vi "Test Run Suite of Several Suites.vi"(8 "error in (no error)":errorcluster, 11 "Test Case In":refnum<class "LUnit Test Suite Tests.lvclass">) -> (0 "error out":errorcluster, 3 "Test Case Out":refnum<class "LUnit Test Suite Tests.lvclass">)   [LabVIEW 2020, in "LUnit Test Suite Tests.lvclass"]
uses:
  LUnit Test Suite Tests.lvclass
  LUnit Test Suite Tests.lvclass/LUnit Test Suite Tests.ctl
  source/LUnit Test Suite.lvclass
  Test Doubles/Test Case Test Double Child/Light Test Case Double.lvclass
  C:/git/astemes-lunit/source/Core/Runnable/Runnable.lvclass
  Test Doubles/Light Test Case Double Copy/Light Test Case Double Copy.lvclass
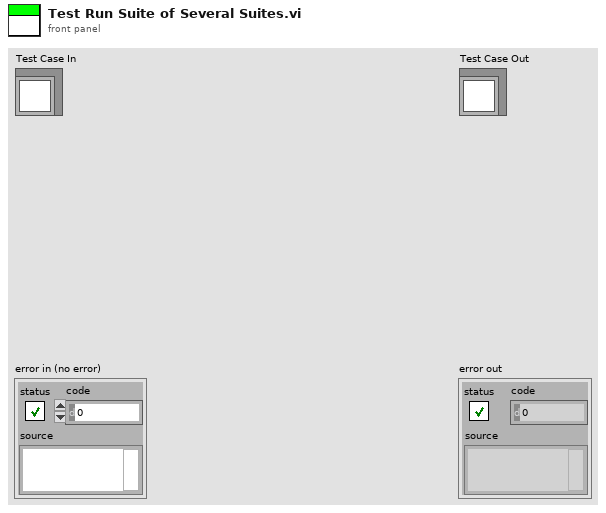
[diagram p1: front panel]
types:
  T1 = typedef "Result.lvlib/Result.ctl" = cluster{"Name":string, "Description":string, "Status":T2, "Result Type":T3, "Execution Time":dbl, "Data":cluster{"Expected":variant, "Actual":variant, "Delta":variant}}
  T2 = typedef "Result.lvlib/Status.ctl" = enum16{"", "Passed", "Failed", "Error", "Skipped", "Setup Error", "Broken", "Teardown Error"}
  T3 = typedef "Result.lvlib/Type.ctl" = enum16{"Test Case", "Test Suite", "Test Run", "Pass", "Fail", "Skip", "Pass if", "Fail if", "Pass if Error", "Fail if Error", "Pass if Equal", "Fail if Equal"}
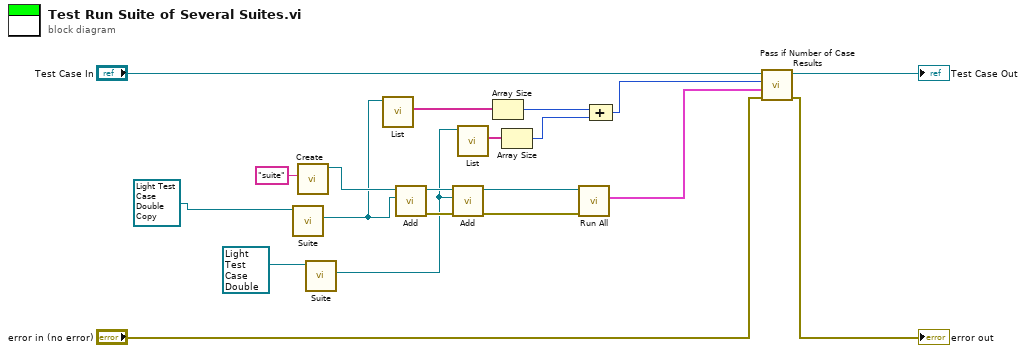
[diagram p0: block diagram]
diagram:
  n1 = call-dynamic "Suite.vi"("LUnit Test Case In"=refnum<class "Light Test Case Double Copy.lvclass"> refnum ("Light Test Case Double Copy.lvclass")) -> ("LUnit Test Suite Out"=w10:refnum<class "LUnit Test Suite.lvclass">)  [unwired: 8 in, 2 out]
  n2 = call "Create.vi"("Suite Name"="suite") -> ("LUnit Test Suite Out"=w11:refnum<class "LUnit Test Suite.lvclass">)  [unwired: 9 in, 1 out]
  n3 = call-dynamic "Suite.vi"("LUnit Test Case In"=refnum<class "Light Test Case Double.lvclass"> refnum ("Light Test Case Double.lvclass")) -> ("LUnit Test Suite Out"=w9:refnum<class "LUnit Test Suite.lvclass">)  [unwired: 8 in, 2 out]
  n4 = call "List.vi"("LUnit Test Suite In"=w10) -> ("List of Runnables"=w6:string[])  [unwired: 9 in, 1 out]
  n5 = call "Add.vi"("Runnable"=w10, "LUnit Test Suite In"=w11) -> ("error out"=w15:errorcluster, "LUnit Test Suite Out"=w14:refnum<class "LUnit Test Suite.lvclass">)  [unwired: 8 in]
  n6 = call "Add.vi"("error in (no error)"=w15, "Runnable"=w9, "LUnit Test Suite In"=w14) -> ("error out"=w16:errorcluster, "LUnit Test Suite Out"=w3:refnum<class "LUnit Test Suite.lvclass">)  [unwired: 7 in]
  n7 = call "List.vi"("LUnit Test Suite In"=w9) -> ("List of Runnables"=w8:string[])  [unwired: 9 in, 1 out]
  n8 = Array Size(array=w6) -> (size(s)=w5:i32)
  n9 = Array Size(array=w8) -> (size(s)=w7:i32)
  n10 = call "Run All.vi"("error in (no error)"=w16, "Runnable In"=w3) -> ("Results"=w1:T1[])  [unwired: 8 in, 1 out]
  n11 = Compound Arithmetic op=ADD(w5, w7) -> (w4:i32)
  n12 = call "Pass if Number of Case Results.vi"("error in (no error)"="error in (no error)", "Results"=w1, "Remaining Results"=w4, "LUnit Test Suite Tests in"="Test Case In") -> ("error out"=→"error out":errorcluster, "LUnit Test Suite Tests out"=→"Test Case Out":refnum<class "LUnit Test Suite Tests.lvclass">)  [unwired: 6 in]
